vi "SubVI_ReadMatGEN_001.vi"(10 "Encoder parameters 2":T1, 11 "1-bit pixmap   in":bool[][](array[boolean])) -> (2 "array of inputs":i32[](array[numeric]), 3 "total #iter":i32)   [LabVIEW 2018]
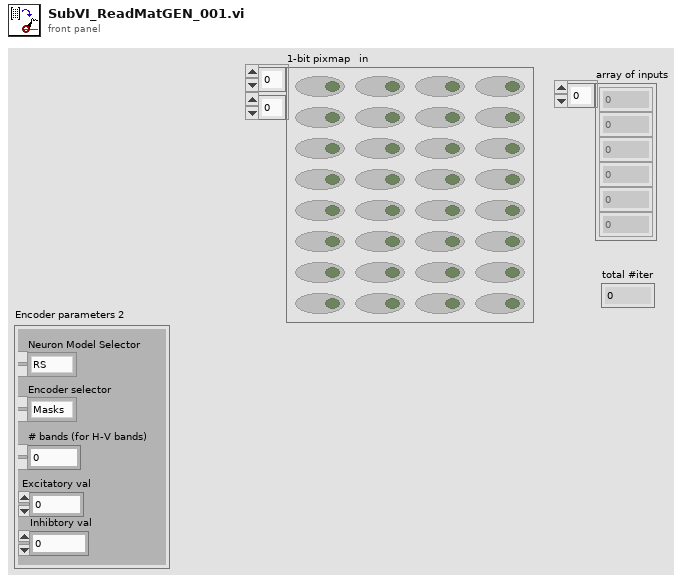
[diagram p1: front panel]
types:
  T1 = cluster{"Encoder selector":enum16{"Masks", "H-V bands", "Simple reading"}, "# bands (for H-V bands)":i32, "Excitatory val":dbl, "Inhibtory val":dbl, "Neuron Model Selector":enum16{"RS", "LTS", "RZ", "TC2", "TC1", "FS", "CH", "IB"}}
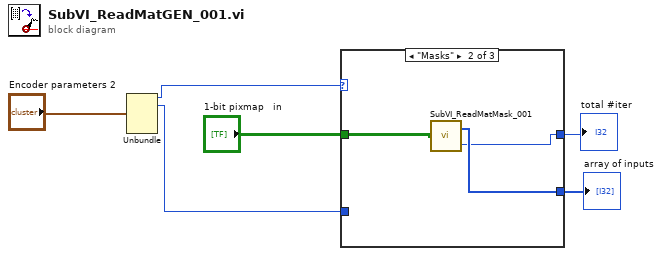
[diagram p0: block diagram]
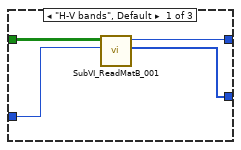
[diagram p2: hidden frame]
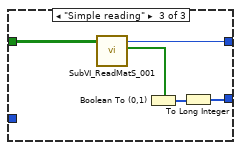
[diagram p3: hidden frame]
diagram:
  n1 = Unbundle("Encoder parameters 2") -> ("Encoder selector"=w3:enum16{"Masks", "H-V bands", "Simple reading"}, "# bands (for H-V bands)"=w2:i32)  [unwired: 3 out]
  n2 = case shown="\"Masks\"" w3 {
    tunnel: "1-bit pixmap   in" -> [w10 w13 w17]
    tunnel: w2 -> [w9 _ _]
    tunnel: [w8 w11 w18] -> w5
    tunnel: [w7 w12 w14] -> w4
    frame "H-V bands", Default {
      n3 = call "SubVI_ReadMatB_001.vi"("# Bands"=w9, "1-bit pixmap   in"=w10) -> ("array of inputs"=w7:i32[], "total #iter"=w8:i32)  [unwired: 8 in]
    }
    frame "Masks" {
      n4 = call "SubVI_ReadMatMask_001.vi"("in IMG"=w13) -> ("Input current"=w12:i32[], "#iter"=w11:i32)
    }
    frame "Simple reading" {
      n5 = call "SubVI_ReadMatS_001.vi"("1-bit pixmap   in"=w17) -> ("array of inputs"=w16:bool[], "total #iter"=w18:i32)  [unwired: 9 in]
      n6 = Boolean To (0,1)(Boolean=w16) -> (0, 1=w15:i16[])
      n7 = To Long Integer(number=w15) -> (32bit integer=w14:i32[])
    }
  }
  "array of inputs" <- w4
  "total #iter" <- w5
